vi "test Position Reset.vi"(8 "error in (no error)":errorcluster, 11 "TestCase in":refnum<class "Engine Simulation IO System Tests.lvclass">) -> (0 "error out":errorcluster, 3 "TestCase out":refnum<class "Engine Simulation IO System Tests.lvclass">)   [LabVIEW 2017, in "Engine Simulation IO System Tests.lvclass"]
uses:
  Engine Simulation IO System Tests.lvclass
  C:/github/niveristand-custom-device-testing-tools/VeriStandTestCase/VeriStandTestCase.lvclass
  <vilib>/NI Veristand/Execution/Workspace/NI VeriStand - Set Single Channel Value.vi
  <vilib>/NI Veristand/Execution/Workspace/NI VeriStand - Get Multiple Channel Values.vi
  <vilib>/addons/_JKI Toolkits/VI Tester/TestCase.llb/TestCase.lvclass
  <vilib>/NI VeriStand/Execution/Workspace/NI_VS Workspace ExecutionAPI.lvlib
  C:/Program Files (x86)/National Instruments/LabVIEW 2017/vi.lib/addons/_JKI Toolkits/VI Tester/TestCase.llb/TestCase.lvclass
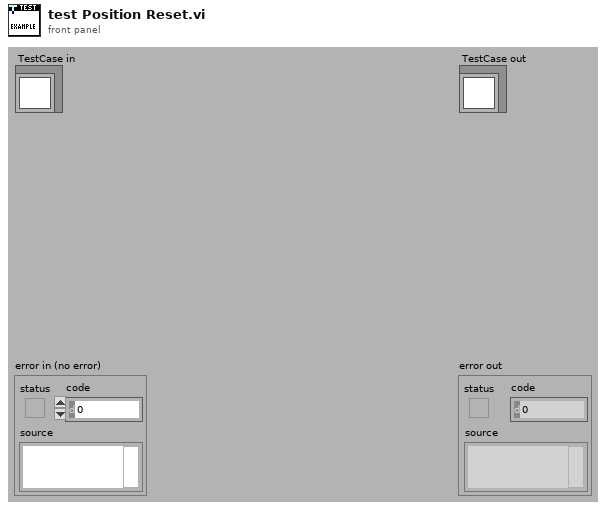
[diagram p1: front panel]
types:
  T1 = typedef "NI_VS Workspace ExecutionAPI.lvlib/WorkspaceAPI.ctl" = refnum<k24>
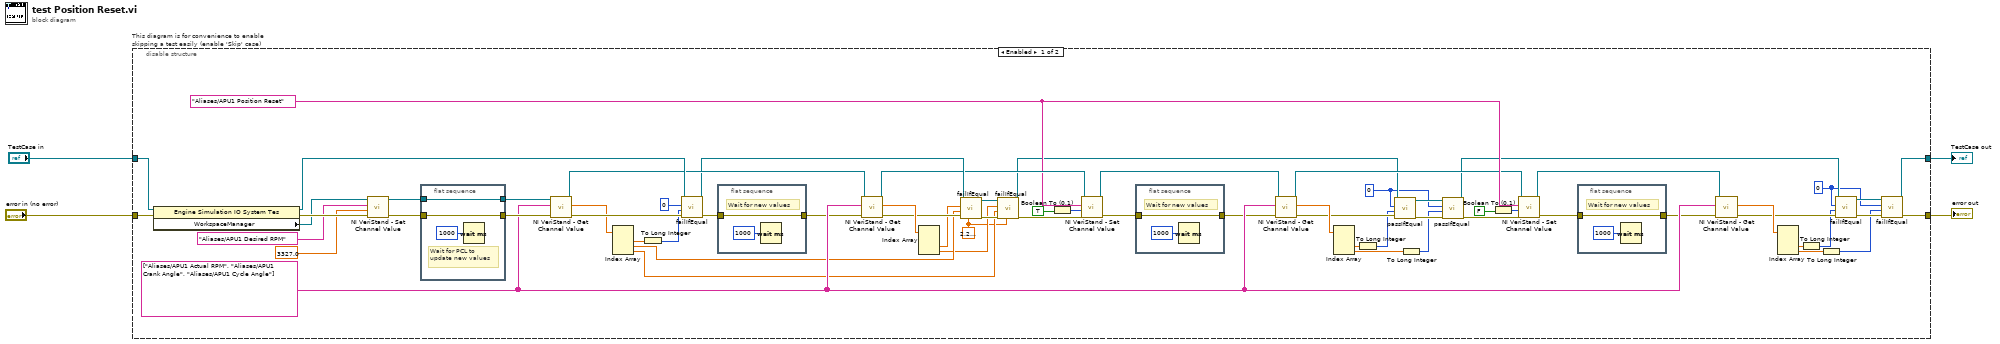
[diagram p0: block diagram]
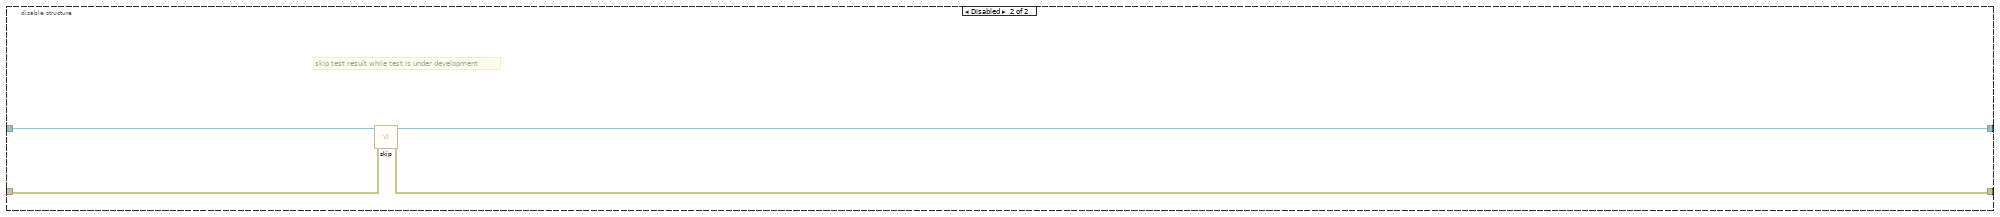
[diagram p2: hidden frame]
diagram:
  n1 = disable-structure "This diagram is for convenience to enable skipping a test easily (enable 'Skip' case)" shown="Enabled" {
    disable-tunnel: "TestCase in" -> [w70 w84]
    disable-tunnel: [w20 w82] -> w1
    disable-tunnel: [w19 w83] -> w3
    disable-tunnel: "error in (no error)" -> [w71 w81]
    frame Enabled {
      w5 = 0 ("32bit integer")
      w12 = 0 ("32bit integer")
      w18 = 2.220446049250313e-16
      w45 = string[] ["Aliases/APU1 Actual RPM", "Aliases/APU1 Crank Angle", "Aliases/APU1 Cycle Angle"]
      w47 = "Aliases/APU1 Position Reset"
      n2 = property class="Engine Simulation IO System Tes"(reference=w70, error in=w71) -> (reference out=w61:refnum<class "Engine Simulation IO System Tests.lvclass">, error out=w69:errorcluster, "WorkspaceManager"=w68:T1)
      n3 = call-poly <vilib>:"NI VeriStand - Set Channel Value.vi"("error in (no error)"=w69, "Value"=3327.0, "Channel"="Aliases/APU1 Desired RPM", "WorkspaceManager in"=w68) -> ("error out"=w65:errorcluster, "WorkspaceManager out"=w64:T1)  [unwired: 6 in]
      n4 = flat-sequence {
        tunnel: w64 -> [w79]
        tunnel: w65 -> [w80]
        tunnel: [w80] -> w63
        tunnel: [w79] -> w62
        frame #0 {
          # "Wait for PCL to\nupdate new values"
          n5 = Wait (ms)(milliseconds to wait=u32 1000) -> ()  [unwired: 1 out]
        }
      }
      n6 = call-poly <vilib>:"NI VeriStand - Get Channel Value.vi"("error in (no error)"=w63, "Channels"=w45, "WorkspaceManager in"=w62) -> ("error out"=w60:errorcluster, "Values"=w57:dbl[], "WorkspaceManager out"=w56:T1)  [unwired: 6 in]
      n7 = Index Array(array=w57) -> (element #1=w17:dbl, element #2=w29:dbl, element #3=w27:dbl)  [unwired: 3 in]
      n8 = To Long Integer(number=w17) -> (32bit integer=w16:i32)
      n9 = call-dynamic "failIfEqual.vi"("error in (no error)"=w60, "y"=w16, "x"=0 ("32bit integer"), "TestCase in"=w61) -> ("error out"=w41:errorcluster, "TestCase out"=w53:refnum<class "Engine Simulation IO System Tests.lvclass">)  [unwired: 6 in]
      n10 = flat-sequence {
        tunnel: w41 -> [w77]
        tunnel: [w77] -> w40
        frame #0 {
          # "Wait for new values"
          n11 = Wait (ms)(milliseconds to wait=u32 1000) -> ()  [unwired: 1 out]
        }
      }
      n12 = call-poly <vilib>:"NI VeriStand - Get Channel Value.vi"("error in (no error)"=w40, "Channels"=w45, "WorkspaceManager in"=w56) -> ("error out"=w54:errorcluster, "Values"=w55:dbl[], "WorkspaceManager out"=w52:T1)  [unwired: 6 in]
      n13 = Index Array(array=w55) -> (element #2=w30:dbl, element #3=w28:dbl)  [unwired: 3 in, 1 out]
      n14 = call-dynamic "failIfEqual.vi"("delta (optional)"=w18, "error in (no error)"=w54, "y"=w29, "x"=w30, "TestCase in"=w53) -> ("error out"=w33:errorcluster, "TestCase out"=w32:refnum<class "Engine Simulation IO System Tests.lvclass">)  [unwired: 5 in]
      n15 = call-dynamic "failIfEqual.vi"("delta (optional)"=w18, "error in (no error)"=w33, "y"=w27, "x"=w28, "TestCase in"=w32) -> ("error out"=w31:errorcluster, "TestCase out"=w25:refnum<class "Engine Simulation IO System Tests.lvclass">)  [unwired: 5 in]
      n16 = Boolean To (0,1)(Boolean=TRUE) -> (0, 1=w58:i16)
      n17 = call-poly <vilib>:"NI VeriStand - Set Channel Value.vi"("error in (no error)"=w31, "Value"=w58, "Channel"=w47, "WorkspaceManager in"=w52) -> ("error out"=w39:errorcluster, "WorkspaceManager out"=w37:T1)  [unwired: 6 in]
      n18 = flat-sequence {
        tunnel: w39 -> [w75]
        tunnel: [w75] -> w38
        frame #0 {
          # "Wait for new values"
          n19 = Wait (ms)(milliseconds to wait=u32 1000) -> ()  [unwired: 1 out]
        }
      }
      n20 = call-poly <vilib>:"NI VeriStand - Get Channel Value.vi"("error in (no error)"=w38, "Channels"=w45, "WorkspaceManager in"=w37) -> ("error out"=w26:errorcluster, "Values"=w51:dbl[], "WorkspaceManager out"=w46:T1)  [unwired: 6 in]
      n21 = Index Array(array=w51) -> (element #2=w14:dbl, element #3=w11:dbl)  [unwired: 3 in, 1 out]
      n22 = To Long Integer(number=w14) -> (32bit integer=w13:i32)
      n23 = call-dynamic "passIfEqual.vi"("error in (no error)"=w26, "y"=w13, "x"=w12, "TestCase in"=w25) -> ("error out"=w23:errorcluster, "TestCase out"=w24:refnum<class "Engine Simulation IO System Tests.lvclass">)  [unwired: 6 in]
      n24 = To Long Integer(number=w11) -> (32bit integer=w10:i32)
      n25 = call-dynamic "passIfEqual.vi"("error in (no error)"=w23, "y"=w10, "x"=w12, "TestCase in"=w24) -> ("error out"=w48:errorcluster, "TestCase out"=w42:refnum<class "Engine Simulation IO System Tests.lvclass">)  [unwired: 6 in]
      n26 = Boolean To (0,1)(Boolean=FALSE) -> (0, 1=w50:i16)
      n27 = call-poly <vilib>:"NI VeriStand - Set Channel Value.vi"("error in (no error)"=w48, "Value"=w50, "Channel"=w47, "WorkspaceManager in"=w46) -> ("error out"=w36:errorcluster, "WorkspaceManager out"=w34:T1)  [unwired: 6 in]
      n28 = flat-sequence {
        tunnel: w36 -> [w73]
        tunnel: [w73] -> w35
        frame #0 {
          # "Wait for new values"
          n29 = Wait (ms)(milliseconds to wait=u32 1000) -> ()  [unwired: 1 out]
        }
      }
      n30 = call-poly <vilib>:"NI VeriStand - Get Channel Value.vi"("error in (no error)"=w35, "Channels"=w45, "WorkspaceManager in"=w34) -> ("error out"=w43:errorcluster, "Values"=w44:dbl[])  [unwired: 6 in, 1 out]
      n31 = Index Array(array=w44) -> (element #2=w9:dbl, element #3=w8:dbl)  [unwired: 3 in, 1 out]
      n32 = To Long Integer(number=w9) -> (32bit integer=w7:i32)
      n33 = To Long Integer(number=w8) -> (32bit integer=w6:i32)
      n34 = call-dynamic "failIfEqual.vi"("error in (no error)"=w43, "y"=w7, "x"=w5, "TestCase in"=w42) -> ("error out"=w22:errorcluster, "TestCase out"=w21:refnum<class "Engine Simulation IO System Tests.lvclass">)  [unwired: 6 in]
      n35 = call-dynamic "failIfEqual.vi"("error in (no error)"=w22, "y"=w6, "x"=w5, "TestCase in"=w21) -> ("error out"=w19:errorcluster, "TestCase out"=w20:refnum<class "Engine Simulation IO System Tests.lvclass">)  [unwired: 6 in]
    }
    frame Disabled {
      # "skip test result while test is under development"
      n36 = call <vilib>:"skip.vi"("error in (no error)"=w81, "TestCase in"=w84) -> ("error out"=w83:errorcluster, "TestCase out"=w82:refnum<class "Engine Simulation IO System Tests.lvclass">)  [unwired: 8 in]
    }
  }
  "error out" <- w3
  "TestCase out" <- w1
